vi "Test External Clock.vi"() -> ()   [LabVIEW 2021]
uses:
  Typedef/Clock Conversion.ctl
  Typedef/Timestamp Pair.ctl
  Typedef/Clock Error Statistics.ctl
  Typedef/Clock History Map.ctl
  Typedef/Clock History.ctl
  Typedef/Clock Conversion Map.ctl
  <vilib>/Platform/TimedLoop/XDataNode/timing_clust.ctl
  <vilib>/Platform/TimedLoop/XDataNode/nitl_modes.ctl
  <vilib>/Platform/TimedLoop/XDataNode/wakeup.ctl
  <vilib>/numeric/Random Number (Range) I64.vi
  System Time/LabVIEW Time to TAI Time.vi
  <vilib>/numeric/sub_Random U32.vi
  SubVIs/Add Error.vi
  Errors/Append Error Location.vi
  <vilib>/Analysis/baseanly.llb/Std Deviation and Variance.vi
  <vilib>/platform/TimedLoop/XDataNode/XDataNode.xnode
  <vilib>/Platform/TimedLoop/XDataNode/XDNodeRunTimeDep.lvlib
  Time_CIF_U.lvlib
panel:
  out "Error Statistics (ns)":T1
  in  "PPM Random Frequency Error":i64=100
  in  "Sample Noise":i64=50000
  out "Clock Conversion Array":T2[](array[typedef])
  out "error out":errorcluster
  out "Conversion error":i64
  out "Result Error (ns)":i64
  out "Error Chart 2":i64(graph)
  in  "stop":bool
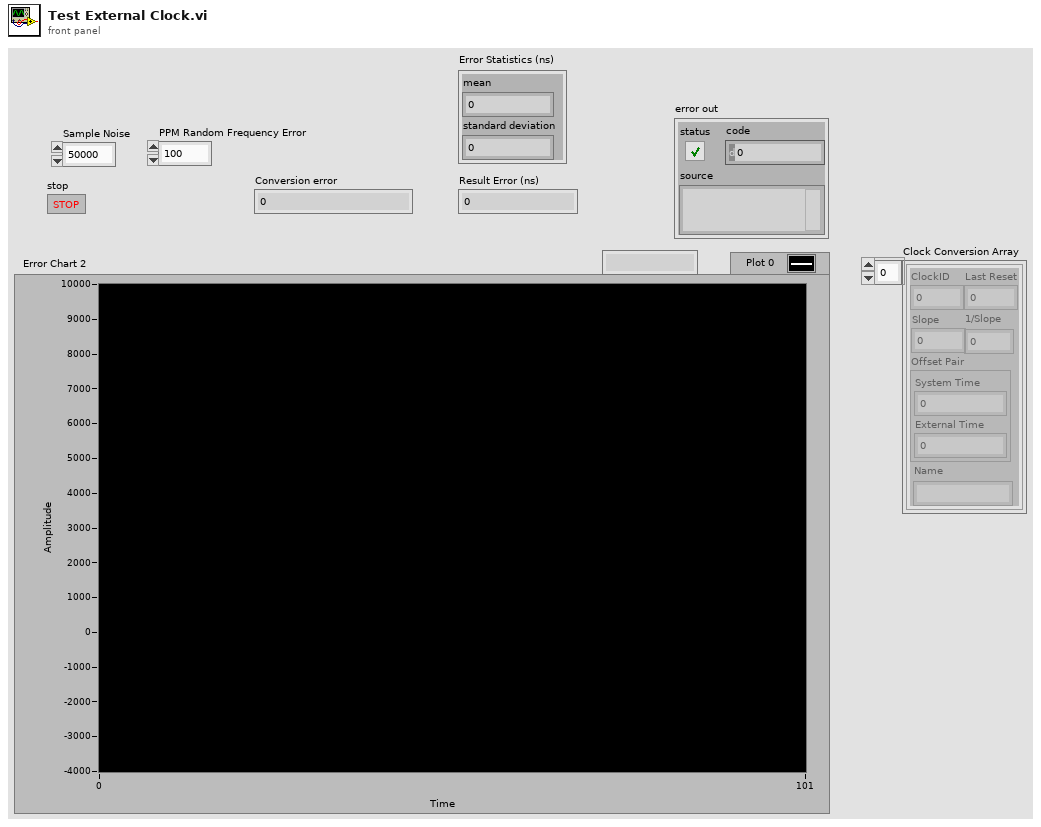
[diagram p1: front panel]
types:
  T1 = typedef "Time_CIF_U.lvlib/Clock Error Statistics.ctl" = cluster{"mean":i64, "standard deviation":i64}
  T2 = typedef "Time_CIF_U.lvlib/Clock Conversion.ctl" = cluster{"ClockID":u8, "Last Reset":i64, "Offset Pair":T3, "Slope":dbl, "1/Slope":dbl, "Name":string}
  T3 = typedef "Time_CIF_U.lvlib/Timestamp Pair.ctl" = cluster{"System Time":i64, "External Time":i64}
  T4 = typedef "Time_CIF_U.lvlib/Clock Conversion Map.ctl" = map{u8, cluster{"Last Reset":i64, "Offset Pair":T3, "Slope":dbl, "1/Slope":dbl}}
  T5 = typedef "Time_CIF_U.lvlib/Clock History Map.ctl" = map{u8, T6}
  T6 = typedef "Time_CIF_U.lvlib/Clock History.ctl" = cluster{"System Clock":i64[], "External Clock":i64[], "Last Reset Time":i64, "slope":dbl, "1/slope":dbl, "Offset Pair":T3, "Name":string}
  T7 = typedef "XDNodeRunTimeDep.lvlib/timing_clust.ctl" = cluster{"Expected End [f-1]":u64, "Actual End [f-1]":u64, "Finished Late? [f-1]":bool, "Expected End [i-1]":u64, "Actual End [i-1]":u64, "Finished Late? [i-1]":bool, "Expected Start [i]":u64, "Actual Start [i]":u64, "Expected Start [f]":u64, "Actual Start [f]":u64, "Source Name":string, "Structure Name":string, "Period":i64, "Deadline":i64, "Offset":i64, "Start":i64, "Priority":i32, "Timeout":i32, "Mode":T8, "Wakeup Reason":T9, "Error":errorcluster, "Source Type":string, "Secondary Source Type":string, "Global End Time":u64, "Global Start Time":u64, "Frame Duration":u64, "Iteration Duration":u64, "Assigned CPU":i32, "I/O Scan Engine Mode":u32}
  T8 = typedef "XDNodeRunTimeDep.lvlib/nitl_modes.ctl" = enum32{"No Change", "Process missed periods, maintain original phase", "Discard missed periods, maintain original phase", "Process missed periods, ignore original phase", "Discard missed periods, ignore original phase"}
  T9 = typedef "XDNodeRunTimeDep.lvlib/wakeup.ctl" = enum32{"Normal", "Aborted", "Asynchronous wakeup", "Timing source error", "Timed loop error", "Timeout"}
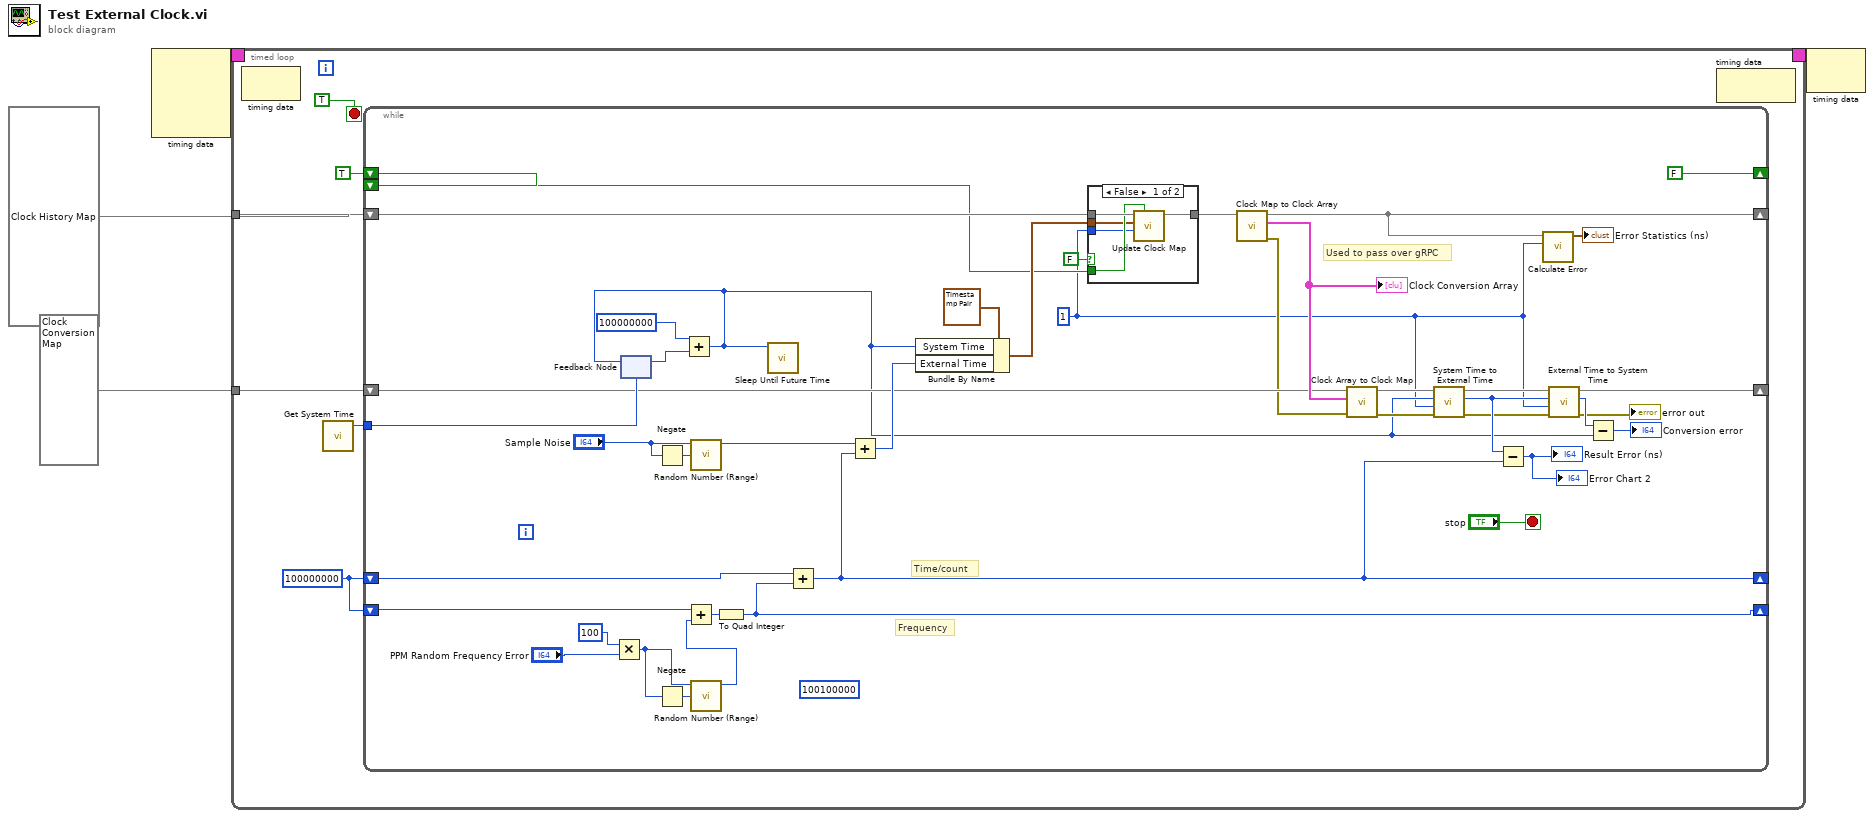
[diagram p0: block diagram]
diagram:
  n1 = node-c288() -> (w4:T7)  [unwired: 4 in]
  n2 = timed-loop {
    timing: w4 -> [_]
    timing-out: [_] -> w3
    tunnel: T5 {} ("Clock History Map in") -> [w8]
    tunnel: T4 {} ("Clock Convert Map out") -> [w6]
    stop <- TRUE stop-if-true
    w5 = i64 100000000 ("y")
    w7 = TRUE
    n3 = node-c288() -> ()  [unwired: 1 in, 1 out]
    n4 = call "Get System Time.vi"() -> ("Time (ns)"=w9:i64)  [unwired: 5 in]
    n5 = while {
      tunnel: w9 -> [w51]
      shift-right: [w13] -> _
      shift-left: w8 -> [w49]
      shift-right: [FALSE] -> _
      shift-left: w7 -> [_]
      shift-left: w7 -> [w45]
      shift-right: [w34] -> _
      shift-left: w6 -> [w33]
      shift-right: [w21] -> _
      shift-left: w5 -> [w22]
      shift-right: [w18] -> _
      shift-left: w5 -> [w20]
      stop <- "stop" stop-if-true
      (unwired) i64 100100000 ("y")
      w12 = u8 1 ("ClockID")
      # "Frequency"
      # "Time/count"
      # "Used to pass over gRPC"
      n6 = Multiply(x=i64 100, y="PPM Random Frequency Error") -> (x*y=w15:i64)
      n7 = feedback #1(w51) -> (w50:i64)
      n8 = Negate(x="Sample Noise") -> (-x=w23:i64)
      n9 = Negate(x=w15) -> (-x=w17:i64)
      n10 = Add(x=i64 100000000 ("y"), y=w50) -> (x+y=w28:i64)
      n11 = feedback-in #1(w28) -> ()
      n12 = call-poly <vilib>:"Random Number (Range).vi"("lower bound (-100)"=w23, "upper bound (100)"="Sample Noise") -> ("number"=w26:i64)  [unwired: 9 in]
      n13 = call-poly <vilib>:"Random Number (Range).vi"("lower bound (-100)"=w17, "upper bound (100)"=w15) -> ("number"=w14:i64)  [unwired: 9 in]
      n14 = Add(x=w20, y=w14) -> (x+y=w25:i64)
      n15 = To Quad Integer(1:w25) -> (0:w18:i64)
      n16 = call "Sleep Until Future Time.vi"("Wake Time (ns)"=w28) -> ()  [unwired: 8 in, 3 out]
      n17 = Add(x=w22, y=w18) -> (x+y=w21:i64)
      n18 = Add(x=w26, y=w21) -> (x+y=w38:i64)
      n19 = Bundle By Name(cluster=T3 {"System Time"=1726494902617542000, "External Time"=44044000000} ("Timestamp Pair"), "System Time"=w28, "External Time"=w38) -> (w47:T3)
      n20 = case shown="False" FALSE {
        tunnel: w49 -> [w57 w58]
        tunnel: w47 -> [w54 _]
        tunnel: [w56 w58] -> w37
        tunnel: w12 -> [w53 _]
        tunnel: w45 -> [w55 _]
        frame False {
          n21 = call "Update Clock Map.vi"("Reset"=w55, "ClockID"=w53, "Timestamp Pair"=w54, "Clock History Map in"=w57) -> ("Clock History Map out"=w56:map{u8, T6})  [unwired: 6 in, 1 out]
        }
        frame True {
        }
      }
      n22 = call "Clock Map to Clock Array.vi"("Clock History Map in"=w37) -> ("error out"=w32:errorcluster, "Clock Conversion Array"=w36:T2[], "Clock History Map out"=w13:T5)  [unwired: 8 in]
      "Clock Conversion Array" <- w36
      n23 = call "Clock Array to Clock Map.vi"("error in (no error)"=w32, "Clock Conversion Array"=w36, "Clock Convert Map in"=w33) -> ("error out"=w31:errorcluster, "Clock Convert Map out"=w35:T4)  [unwired: 7 in]
      n24 = call "System Time to External Time.vi"("error in (no error)"=w31, "ClockID"=w12, "System Time"=w28, "Clock Convert Map in"=w35) -> ("error out"=w30:errorcluster, "External Time"=w43:i64, "Clock Convert Map out"=w44:T4)  [unwired: 4 in, 1 out]
      n25 = Subtract(x=w43, y=w21) -> (x-y=→"Result Error (ns)" →"Error Chart 2":i64)
      n26 = call "Calculate Error.vi"("ClockID"=w12, "Clock History Map in"=w13) -> ("Error Statistics (ns)"=→"Error Statistics (ns)":T1)  [unwired: 8 in, 1 out]
      n27 = call "External Time to System Time.vi"("error in (no error)"=w30, "ClockID"=w12, "External Time"=w43, "Clock Convert Map in"=w44) -> ("error out"=→"error out":errorcluster, "System Time"=w42:i64, "Clock Convert Map out"=w34:T4)  [unwired: 4 in, 1 out]
      n28 = Subtract(x=w42, y=w28) -> (x-y=→"Conversion error":i64)
    }
    n29 = node-c288() -> ()  [unwired: 1 in, 1 out]
  }
  n30 = node-c288(w3) -> ()  [unwired: 1 out]
